vi "LastTestPassedGreen.vi"(8 "error in (no error)":errorcluster, 9 "Message":string, 10 "Delay msecs (1000)":u32=1000, 11 "Wait for key press? (n)":bool) -> (0 "error out":errorcluster)   [LabVIEW 2013]
panel:
  in  "String":string
  # "Last test passed"
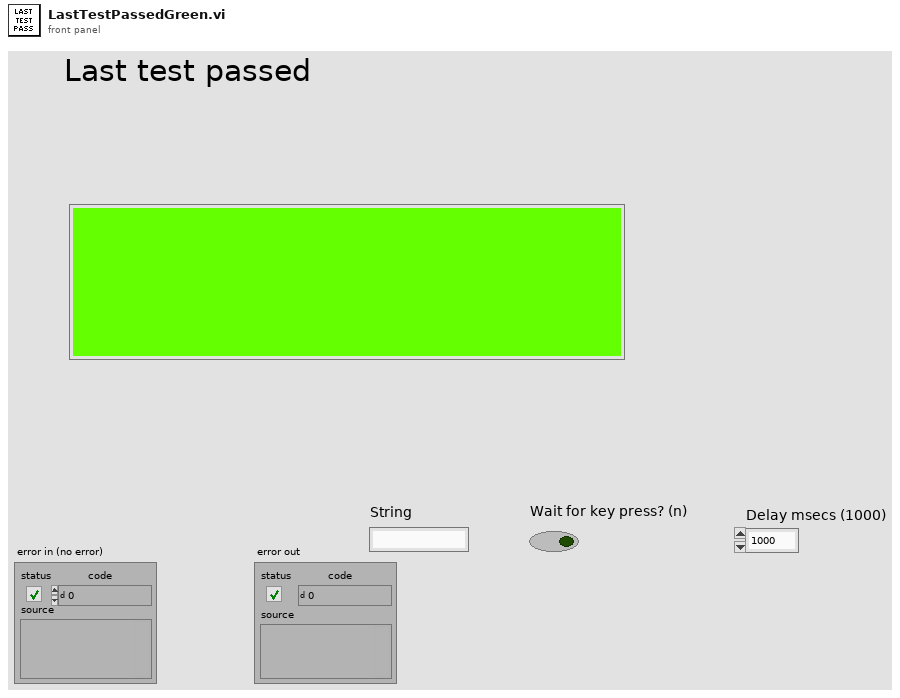
[diagram p1: front panel]
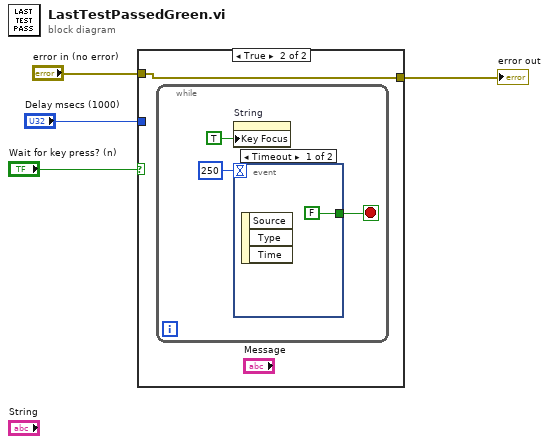
[diagram p0: block diagram]
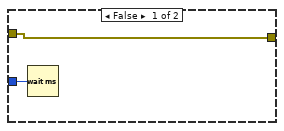
[diagram p2: hidden frame]
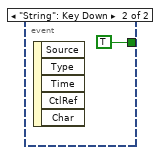
[diagram p3: hidden frame]
diagram:
  n1 = case shown="True" "Wait for key press? (n)" {
    tunnel: "Delay msecs (1000)" -> [w6 _]
    tunnel: "error in (no error)" -> [w5 w7]
    tunnel: [w5 w7] -> w1
    frame False {
      n2 = Wait (ms)(milliseconds to wait=w6) -> ()  [unwired: 1 out]
    }
    frame True {
      n3 = while {
        stop <- w8 stop-if-true
        n4 = property on="String" class="Str"("Key Focus"=TRUE) -> ()  [unwired: 2 in, 2 out]
        n5 = event shown="[0] Timeout" {
          selector: _ -> [_ _]
          dyn-events: _ -> [_ _]
          timeout: 250 -> [_ _]
          tunnel: [FALSE TRUE] -> w8
          event Timeout {
            n6 = event-data() -> ()  [unwired: 1 in, 3 out]
          }
          event "String": Key Down {
            n7 = event-data() -> ()  [unwired: 1 in, 5 out]
          }
        }
      }
    }
  }
  "error out" <- w1
